vi "EngineMain.vi"() -> ()   [LabVIEW 2013]
uses:
  EngineController.ctl
panel:
  out "Engine States":T1
  in  "stop":bool
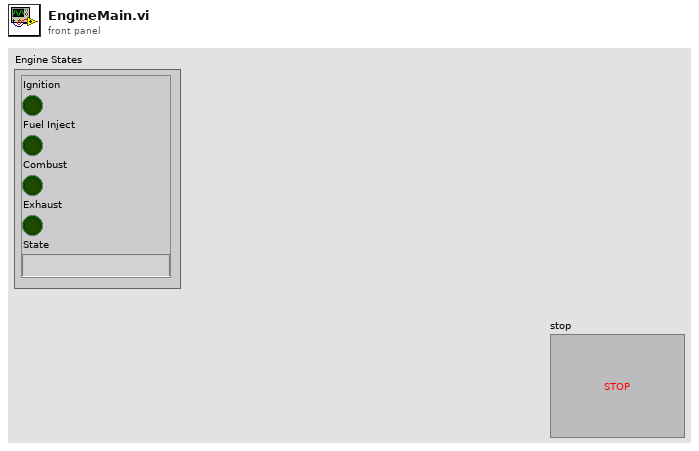
[diagram p1: front panel]
types:
  T1 = cluster{"Ignition":bool, "Fuel Inject":bool, "Combust":bool, "Exhaust":bool, "State":string}
  T2 = typedef "EngineController.ctl" = enum16{"Ignite", "Fuel Inject", "Combust", "Exhaust", "Stop"}
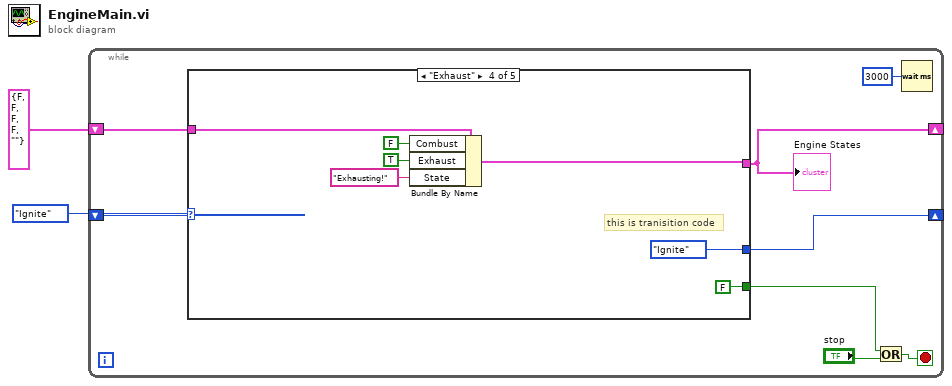
[diagram p0: block diagram]
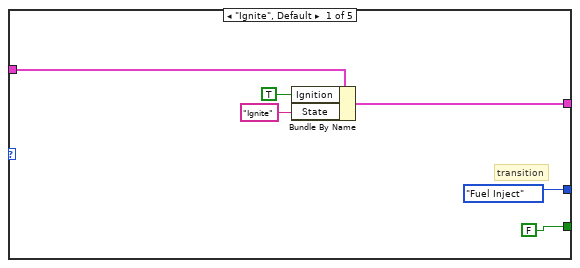
[diagram p2: hidden frame]
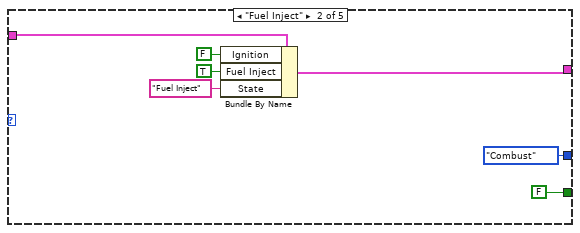
[diagram p3: hidden frame]
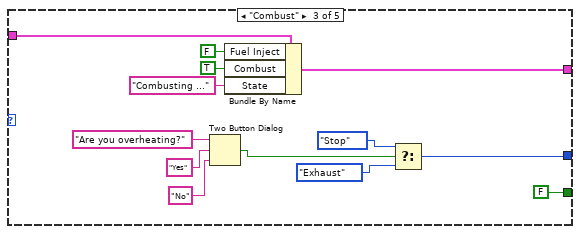
[diagram p4: hidden frame]
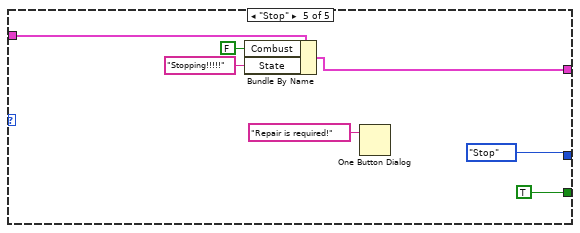
[diagram p5: hidden frame]
diagram:
  n1 = while {
    shift-right: [w3] -> _
    shift-left: EngineController."Ignite" ("Enum") -> [w10]
    shift-right: [w7] -> _
    shift-left: T1 {"Ignition"=FALSE, "Fuel Inject"=FALSE, "Combust"=FALSE, "Exhaust"=FALSE, "State"=""} ("Engine States 2") -> [w8]
    stop <- w6 stop-if-true
    n2 = case shown="\"Exhaust\"" w10 {
      tunnel: w8 -> [w16 w23 w33 w40 w50]
      tunnel: [w15 w19 w32 w39 w45] -> w7
      tunnel: [FALSE FALSE FALSE FALSE TRUE] -> w4
      tunnel: [EngineController."Fuel Inject" ("Enum") EngineController."Combust" ("Enum") w24 EngineController."Ignite" ("Enum") EngineController."Stop" ("Enum")] -> w3
      frame "Ignite", Default {
        # "transition"
        n3 = Bundle By Name(cluster=w16, "Ignition"=TRUE, "State"="Ignite") -> (w15:T1)
      }
      frame "Fuel Inject" {
        n4 = Bundle By Name(cluster=w23, "Ignition"=FALSE, "Fuel Inject"=TRUE, "State"="Fuel Inject") -> (w19:T1)
      }
      frame "Combust" {
        n5 = Two Button Dialog(message="Are you overheating?", 1:"No" ("F button name (\"Cancel\")"), 2:"Yes" ("T button name (\"OK\")")) -> (T button?=w28:bool)
        n6 = Bundle By Name(cluster=w33, "Fuel Inject"=FALSE ("Ignition"), "Combust"=TRUE ("Fuel Inject"), "State"="Combusting ...") -> (w32:T1)
        n7 = Select(t=EngineController."Stop" ("Enum"), s=w28, f=EngineController."Exhaust" ("Enum")) -> (s? t:f=w24:T2)
      }
      frame "Exhaust" {
        # "this is tranisition code"
        n8 = Bundle By Name(cluster=w40, "Combust"=FALSE ("Ignition"), "Exhaust"=TRUE ("Fuel Inject"), "State"="Exhausting!") -> (w39:T1)
      }
      frame "Stop" {
        n9 = Bundle By Name(cluster=w50, "Combust"=FALSE, "State"="Stopping!!!!!") -> (w45:T1)
        n10 = One Button Dialog(message="Repair is required!") -> ()  [unwired: 1 in, 1 out]
      }
    }
    "Engine States" <- w7
    n11 = Or(x=w4, y="stop") -> (x .or. y?=w6:bool)
    n12 = Wait (ms)(milliseconds to wait=u32 3000) -> ()  [unwired: 1 out]
  }
